vi "Check if within limits.vi"(8 "error in (no error)":errorcluster, 10 "Position array in":dbl[](array[numeric]), 11 "StageSPIM in":refnum<class "StageSPIM.lvclass">) -> (0 "error out":errorcluster, 1 "coerced?":bool[](array[boolean]), 2 "Approved postion array":dbl[](array[numeric]), 3 "StageSPIM out":refnum<class "StageSPIM.lvclass">, 4 "one axis coerced?":bool)   [LabVIEW 2012, in "StageSPIM.lvclass"]
uses:
  StageSPIM.lvclass
  StageSPIM.lvclass/StageSPIM.ctl
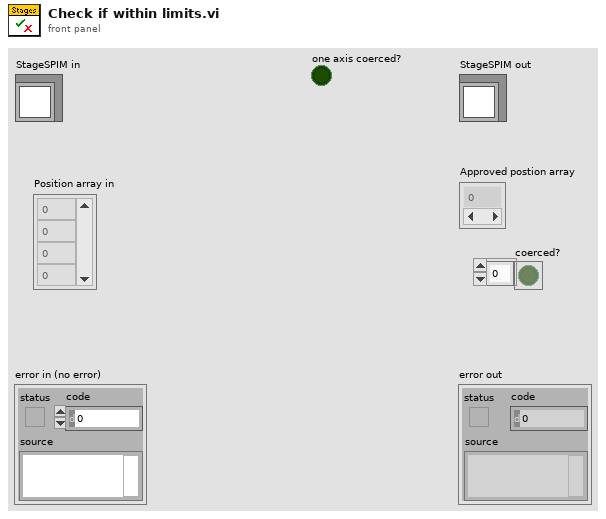
[diagram p1: front panel]
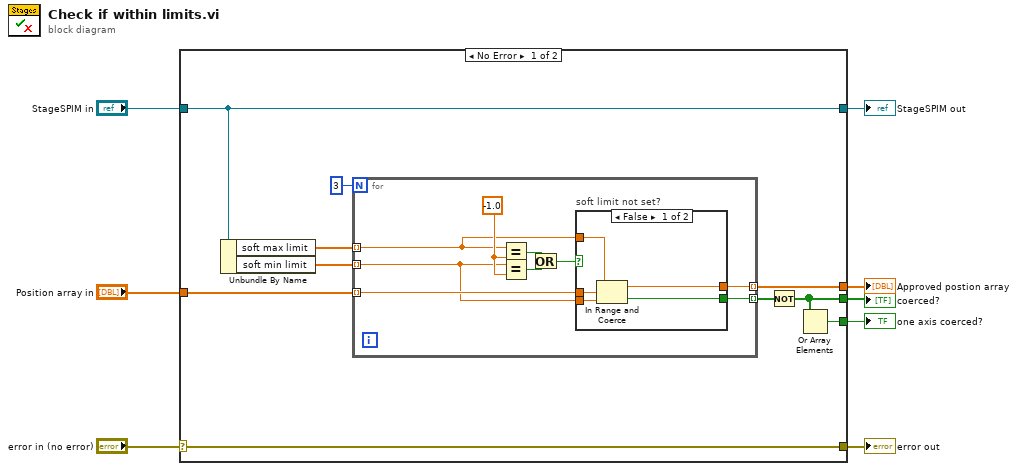
[diagram p0: block diagram]
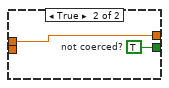
[diagram p2: hidden frame]
diagram:
  n1 = case shown="No Error" "error in (no error)" {
    selector: "error in (no error)" -> [w18 w36]
    tunnel: [w18 w36] -> w7
    tunnel: [w17 w35] -> w5
    tunnel: "StageSPIM in" -> [w17 w35]
    tunnel: "Position array in" -> [w15 _]
    tunnel: [w12 _] -> w3
    tunnel: [w10 _] -> w2
    tunnel: [w9 _] -> w1
    frame No Error {
      n2 = Unbundle By Name(w17) -> ("soft max limit"=w13:dbl[], "soft min limit"=w14:dbl[])
      n3 = for {
        N: 3 -> [_]
        tunnel: w15 -> [w27] mode=indexing
        tunnel: w14 -> [w21] mode=indexing
        tunnel: w13 -> [w22] mode=indexing
        tunnel: [w20] -> w12 mode=indexing
        tunnel: [w19] -> w11 mode=indexing
        w26 = -1.0 ("y")
        n4 = Equal?(x=w22, y=w26) -> (x = y?=w23:bool)
        n5 = Equal?(x=w21, y=w26) -> (x = y?=w24:bool)
        n6 = Or(x=w23, y=w24) -> (x .or. y?=w25:bool)
        n7 = case "soft limit not set?" shown="False" w25 {
          tunnel: w27 -> [w32 w34]
          tunnel: w22 -> [w31 _]
          tunnel: w21 -> [w30 _]
          tunnel: [w29 w34] -> w20
          tunnel: [w28 w33] -> w19
          frame False {
            n8 = In Range and Coerce(upper limit=w31, x=w32, lower limit=w30) -> (coerced(x)=w29:dbl, In Range?=w28:bool)
          }
          frame True {
            w33 = TRUE  # not coerced?
          }
        }
      }
      n9 = Not(x=w11) -> (.not. x?=w10:bool[])
      n10 = Or Array Elements(Boolean array=w10) -> (logical OR=w9:bool)
    }
    frame Error {
    }
  }
  "error out" <- w7
  "StageSPIM out" <- w5
  "Approved postion array" <- w3
  "coerced?" <- w2
  "one axis coerced?" <- w1
